vi "WebCam.CreateCaptureWindowA.vi"(0 "Handle":i32, 5 "NID":i32, 7 "Rect":T1, 11 "ErrorIn":errorcluster) -> (4 "HandleOut":i32, 15 "ErrorOut":errorcluster)   [LabVIEW 2021]
uses:
  avicap32.dll
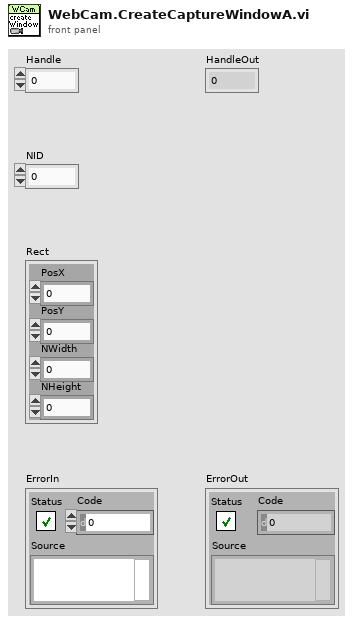
[diagram p1: front panel]
types:
  T1 = cluster{"PosX":i32, "PosY":i32, "NWidth":i32, "NHeight":i32}
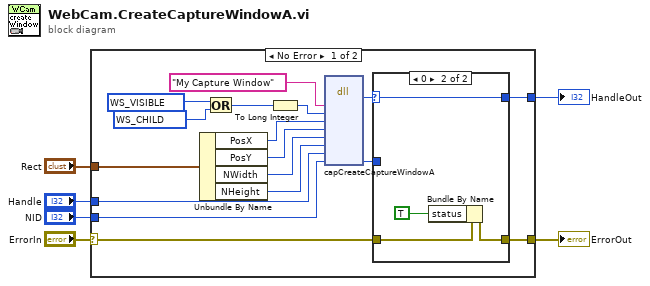
[diagram p0: block diagram]
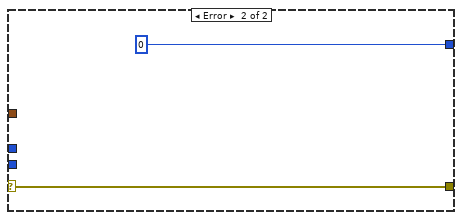
[diagram p3: hidden frame]
diagram:
  n1 = case shown="No Error" "ErrorIn" {
    selector: "ErrorIn" -> [w23 w31]
    tunnel: "Handle" -> [w21 _]
    tunnel: [w17 0] -> w3
    tunnel: "NID" -> [w20 _]
    tunnel: [w22 w31] -> w5
    tunnel: "Rect" -> [w12 _]
    frame No Error {
      w15 = u32 1073741824 items=["WS_CHILD"=1073741824, "WS_VISIBLE"=268435456, "SWP_NOMOVE"=2, "SWP_NOSIZE"=1, "SWP_NOZORDER"=4] ("Ring")
      w16 = u32 268435456 items=["WS_CHILD"=1073741824, "WS_VISIBLE"=268435456, "SWP_NOMOVE"=2, "SWP_NOSIZE"=1, "SWP_NOZORDER"=4] ("Ring")
      n2 = Unbundle By Name(w12) -> ("PosX"=w11:i32, "PosY"=w10:i32, "NWidth"=w9:i32, "NHeight"=w8:i32)
      n3 = Or(x=w16, y=w15) -> (x .or. y?=w14:u32)
      n4 = To Long Integer(number=w14) -> (32bit integer=w13:i32)
      n5 = dll-call lib="avicap32.dll" fn="capCreateCaptureWindowA"("lpszWindowName"="My Capture Window", "dwStyle"=w13, "x"=w11, "y"=w10, "nWidth"=w9, "nHeight"=w8, "hWndParent"=w21, "nID"=w20) -> (w18:i32, "nID"=w7:i32)  [unwired: 10 in, 2 out]
      n6 = case shown="0" w18 {
        selector: w18 -> [w24 w27]
        tunnel: [w24 w27] -> w17
        tunnel: w23 -> [w25 w29]
        tunnel: [w25 w28] -> w22
        tunnel: w7 -> [_ _]
        frame Default {
        }
        frame 0 {
          n7 = Bundle By Name(cluster=w29, "status"=TRUE) -> (w28:errorcluster)
        }
      }
    }
    frame Error {
    }
  }
  "HandleOut" <- w3
  "ErrorOut" <- w5
